vi "correction_data_starter.vi"() -> ()   [LabVIEW 2020]
uses:
  CasaoManagerGeneralSpecifications.ctl
  General dimensions definition.ctl
  Point2D.ctl
  Point2Df.ctl
  WavefrontCorrector.lvclass
  Camera.lvclass
  CorrectionDataManager.lvclass
  Image.lvclass
  InteractionMatrixAcquisitionParameters.ctl
  HasoSlopes.lvclass
  Data alignment enum.ctl
  InteractionMatrixToCommandMatrixParameters.ctl
panel:
  out "Camera Image (2N)":u32[][](graph)
  in  "Start Acq":bool
  out "Camera Image (2N+1)":u32[][](graph)
  in  "number of images to sum":u32=1
  in  "Exposure time (us)":i32=1000
  out "# of valid actuators":u32
  out "Singular values":dbl[](graph)
  in  "Correction data file name":string="Data\\data_correction_manager_example.aomi"
  in  "WavefrontCorrector Configuration file path":path
  out "error out":errorcluster
  out "Informations extracted \nfrom configuration files":T1 caption="Informations extracted from configuration files"
  in  "Haso configuration file path":path
  # "This example is Hardware-dependant, \nplease use your own Haso and corrector configuration file and acquisition system"
  # "Acquisition parameters"
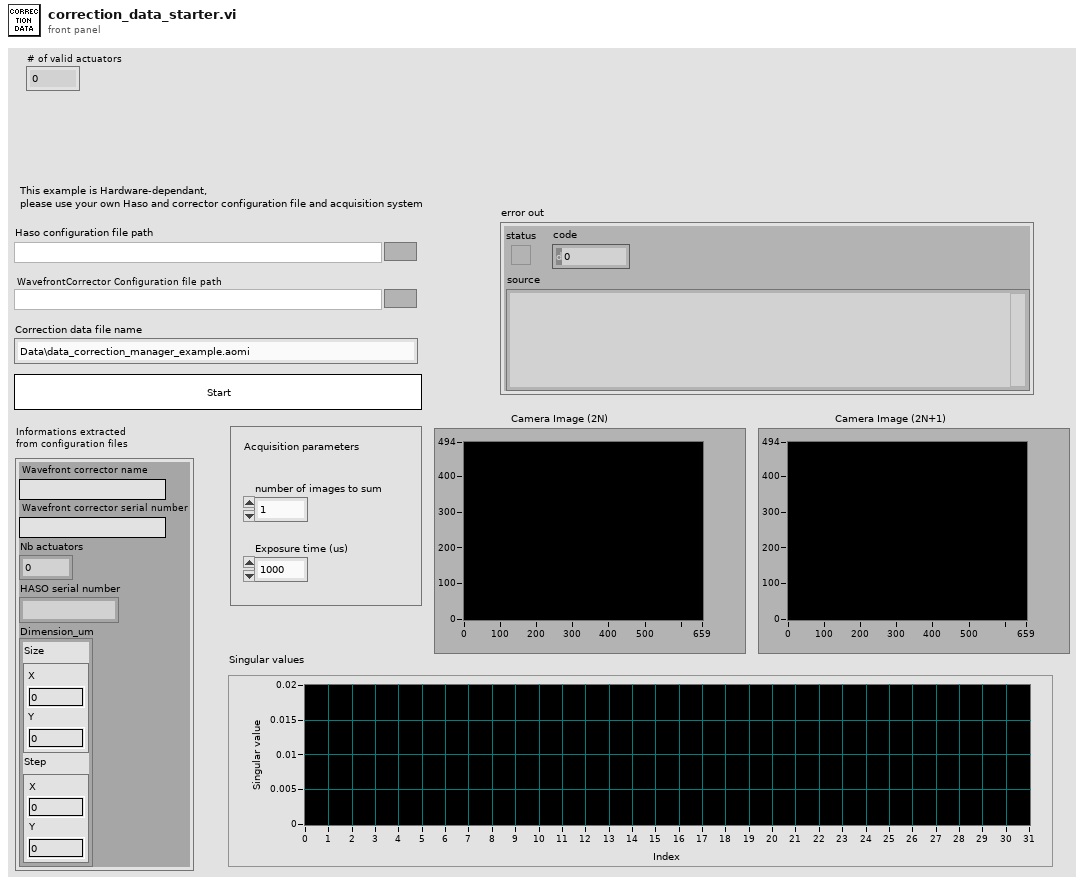
[diagram p1: front panel]
types:
  T1 = typedef "CasaoManagerGeneralSpecifications.ctl" = cluster{"Wavefront corrector name":string, "Wavefront corrector serial number":string, "Nb actuators":i32, "HASO serial number":string, "Dimension_um":T2}
  T2 = typedef "General dimensions definition.ctl" = cluster{"Size":T3, "Step":T4}
  T3 = typedef "Point2D.ctl" = cluster{"X":u32, "Y":u32}
  T4 = typedef "Point2Df.ctl" = cluster{"X":sgl, "Y":sgl}
  T5 = typedef "InteractionMatrixAcquisitionParameters.ctl" = cluster{"Push - Pull value":sgl}
  T6 = typedef "Data alignment enum.ctl" = enum16{"8", "16", "32"}
  T7 = typedef "InteractionMatrixToCommandMatrixParameters.ctl" = cluster{"Number of kept modes":i32, "Tilt filtering":bool}
  T8 = typedef "Wavefront Corrector states - ONE.ctl" = cluster{"Max":sgl, "Min":sgl, "Validity":enum16{"valid", "fixed", "invalid"}, "Fixed_Position":sgl}
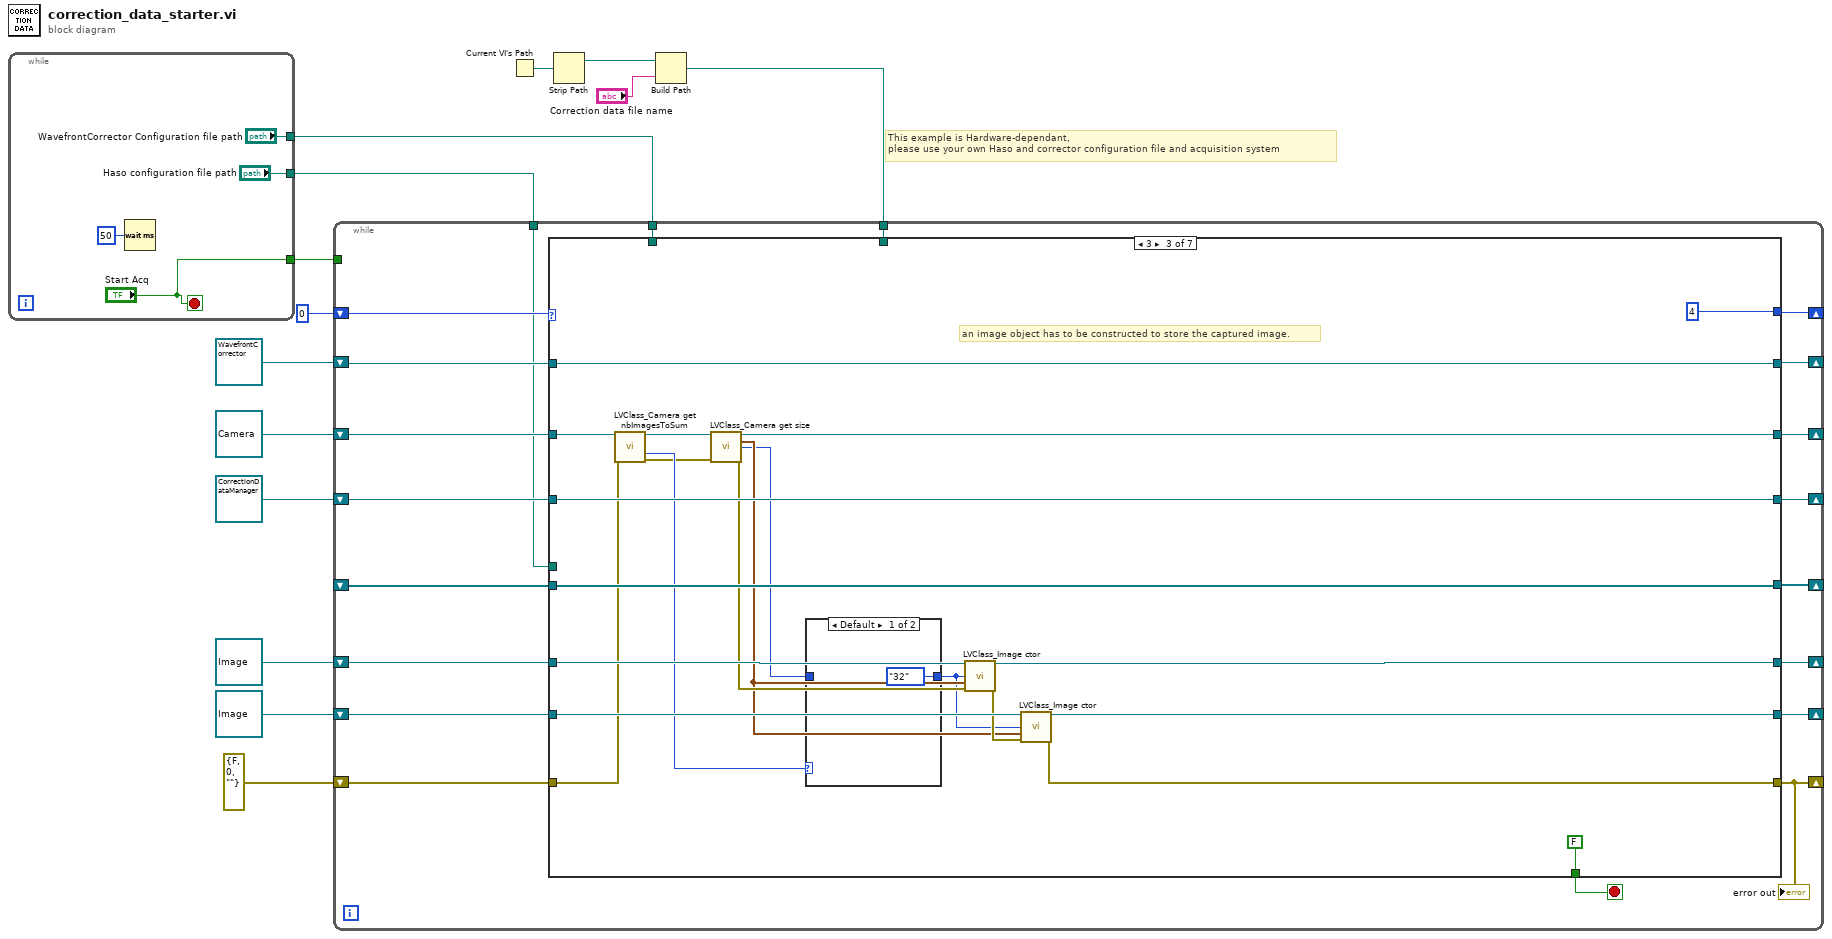
[diagram p0: block diagram]
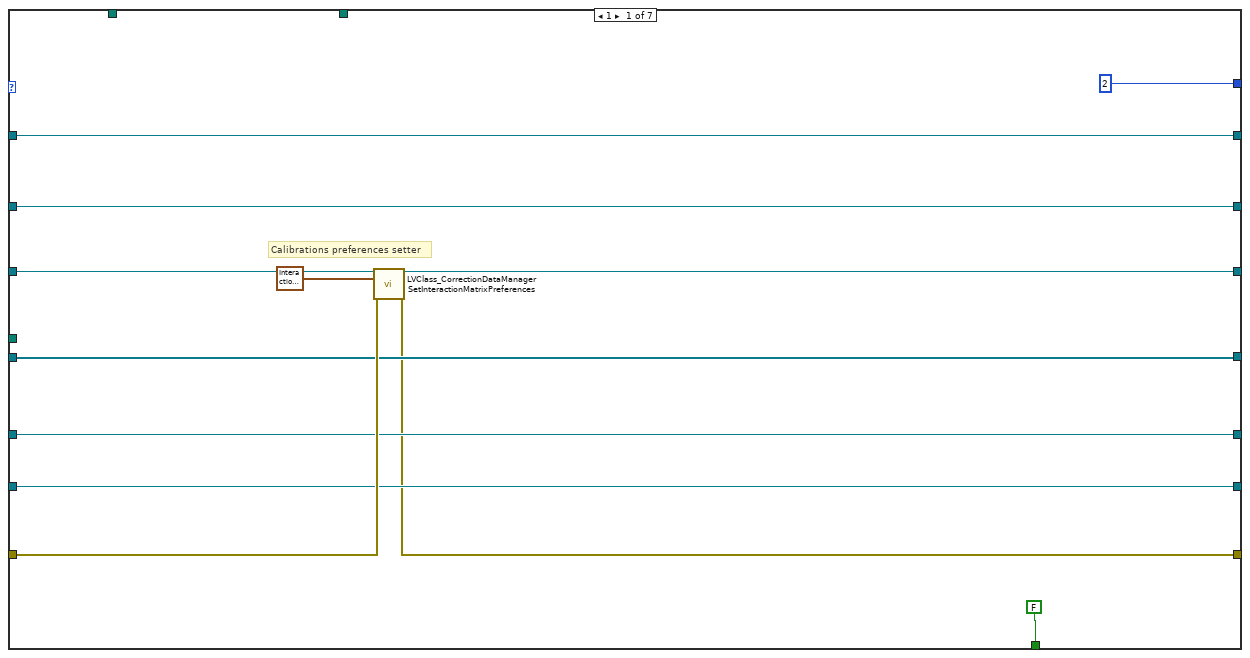
[diagram p2: hidden frame]
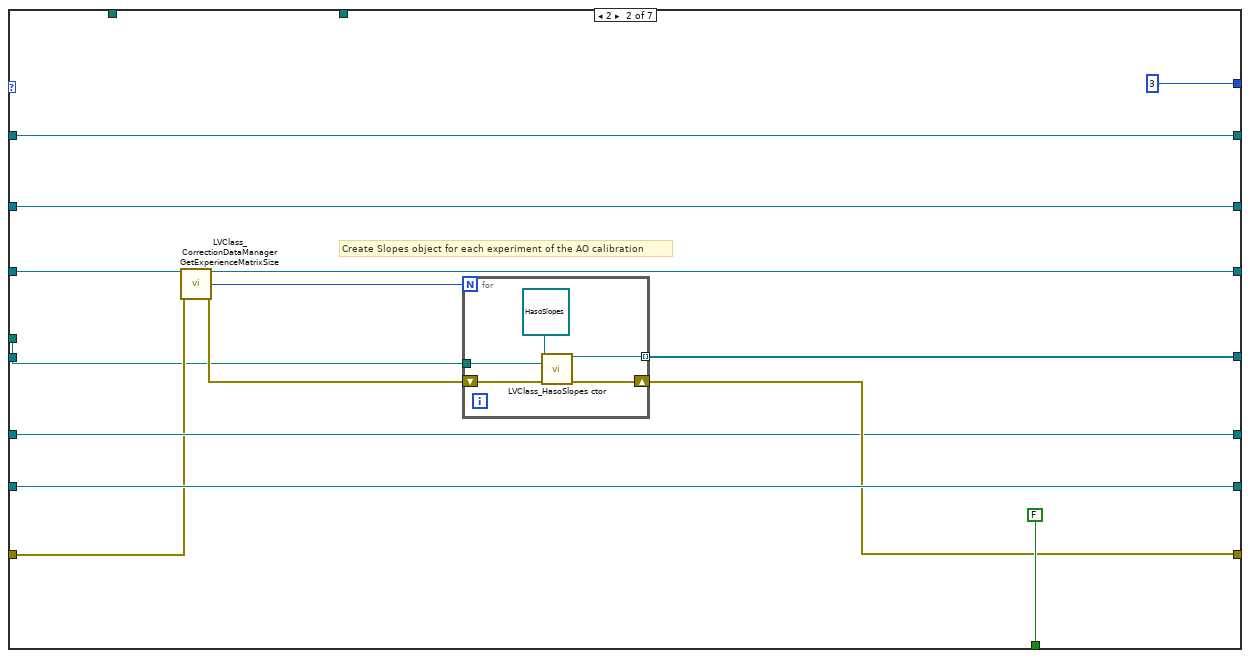
[diagram p3: hidden frame]
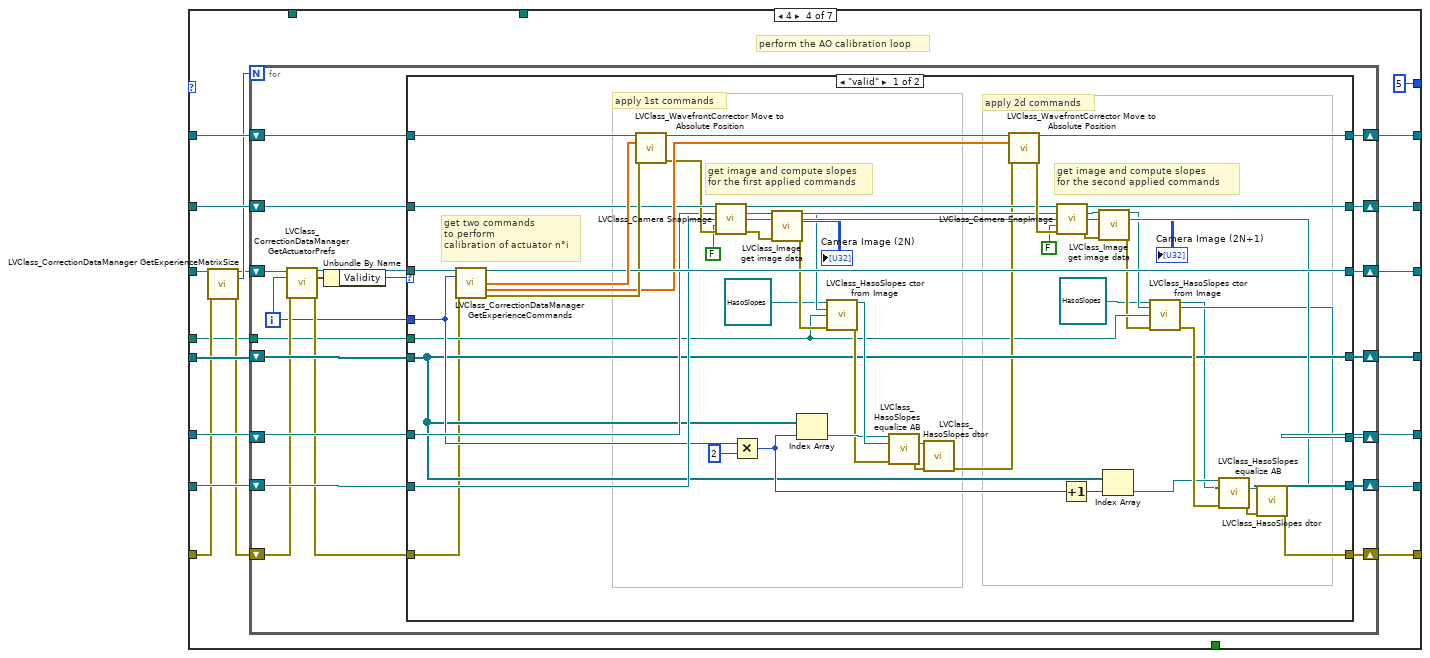
[diagram p5: hidden frame]
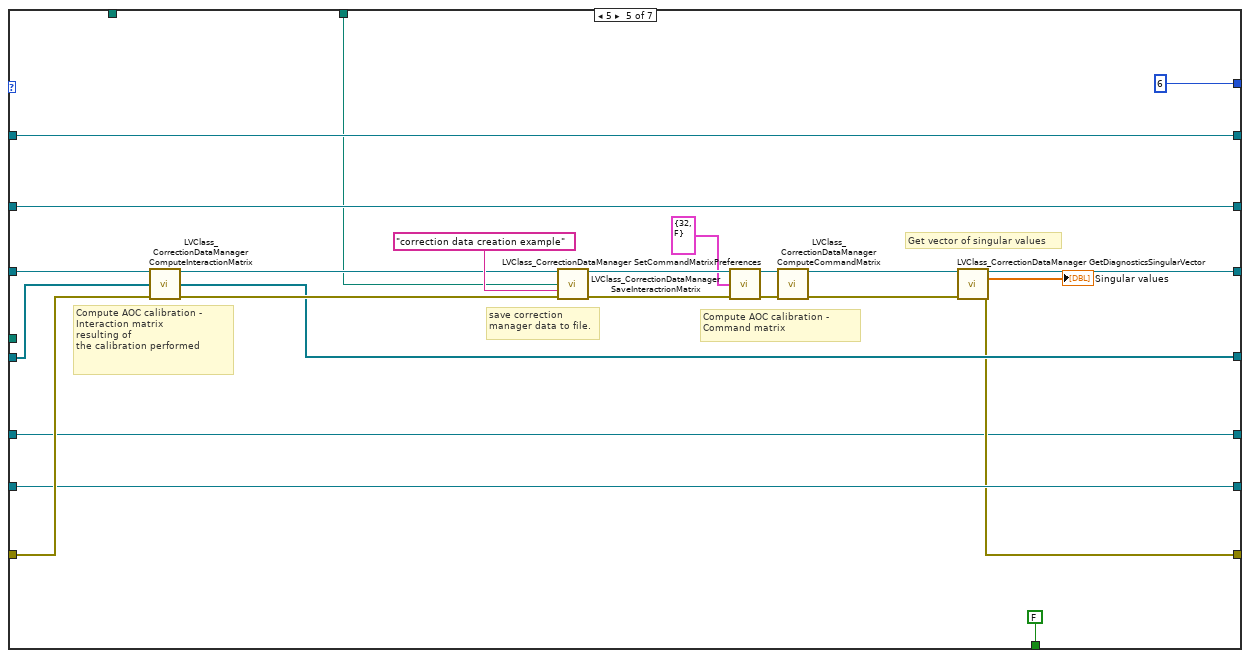
[diagram p7: hidden frame]
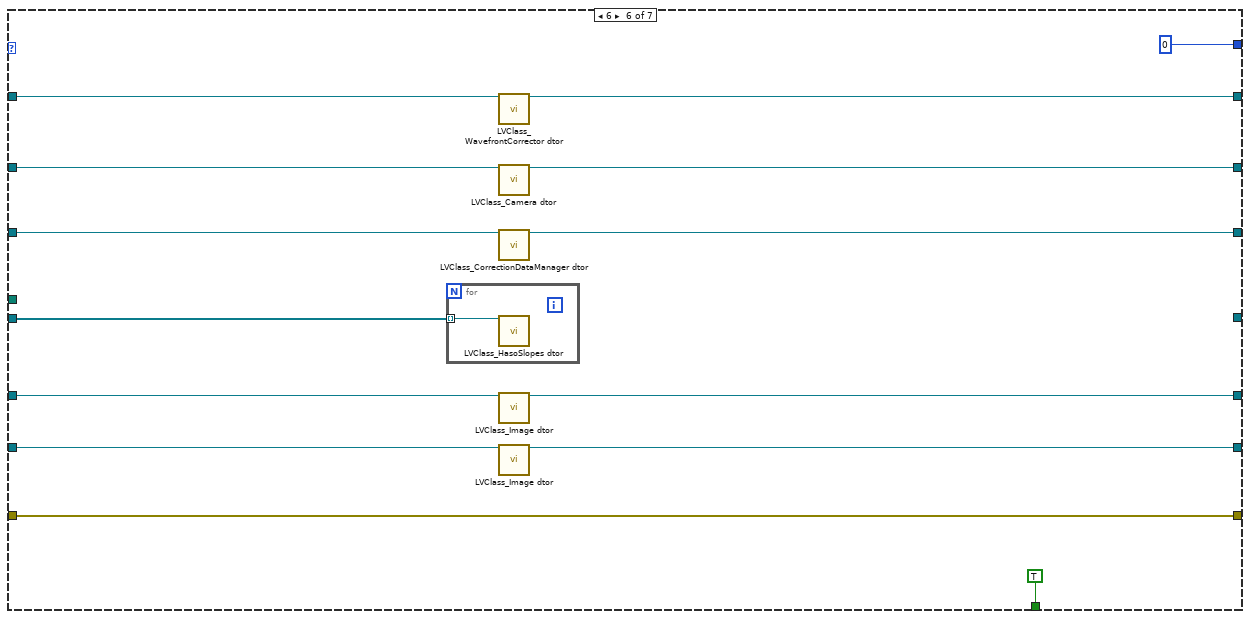
[diagram p8: hidden frame]
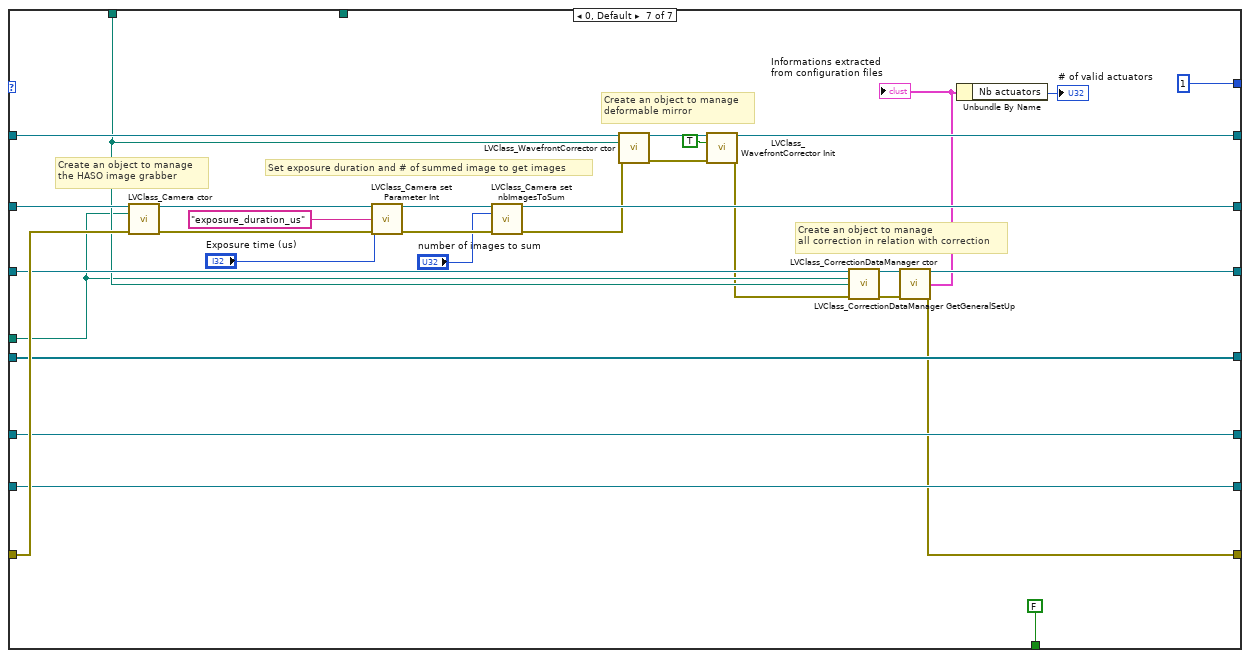
[diagram p9: hidden frame]
diagram:
  # "This example is Hardware-dependant, \nplease use your own Haso and corrector configuration file and acquisition system"
  n1 = while {
    tunnel: ["Start Acq"] -> w8
    tunnel: ["Haso configuration file path"] -> w2
    tunnel: ["WavefrontCorrector Configuration file path"] -> w1
    stop <- "Start Acq" stop-if-true
    n2 = Wait (ms)(milliseconds to wait=u32 50) -> ()  [unwired: 1 out]
  }
  n3 = Current VI's Path() -> (path=w5:path)
  n4 = Strip Path(path=w5) -> (stripped path=w7:path)  [unwired: 1 out]
  n5 = Build Path(base path=w7, name or relative path="Correction data file name") -> (appended path=w4:path)
  n6 = while {
    shift-right: [w30] -> _
    shift-left: refnum<class "WavefrontCorrector.lvclass"> refnum ("WavefrontCorrector in") -> [w32]
    shift-right: [w28] -> _
    shift-left: refnum<class "Camera.lvclass"> refnum ("Camera") -> [w35]
    shift-right: [w29] -> _
    shift-left: refnum<class "CorrectionDataManager.lvclass"> refnum ("CorrectionDataManager in") -> [w31]
    shift-right: [w25] -> _
    shift-left: refnum<class "Image.lvclass"> refnum ("Image in") -> [w27]
    shift-right: [w37] -> _
    shift-left: 0 -> [w38]
    shift-right: [w23] -> _
    shift-left: errorcluster {"status"=FALSE, "code"=0, "source"=""} ("error out") -> [w34]
    tunnel: w1 -> [w33]
    tunnel: w2 -> [w19]
    shift-right: [w26] -> _
    shift-left: _ -> [w24]
    shift-right: [w21] -> _
    shift-left: refnum<class "Image.lvclass"> refnum ("Image out") -> [w22]
    tunnel: w8 -> [_]
    tunnel: w4 -> [w20]
    stop <- w36 stop-if-true
    n7 = case shown="3" w38 {
      tunnel: [2 3 4 5 6 0 1] -> w37
      tunnel: [FALSE FALSE FALSE _ FALSE TRUE FALSE] -> w36
      tunnel: w35 -> [w43 w60 w76 w104 w193 w224 w256]
      tunnel: [w39 w58 w86 w105 w191 w214 w230] -> w23
      tunnel: w34 -> [w46 w55 w73 w95 w208 w214 w255]
      tunnel: w33 -> [_ _ _ _ _ _ w252]
      tunnel: w32 -> [w44 w61 w84 w110 w194 w223 w254]
      tunnel: w19 -> [_ w51 _ w93 _ _ w249]
      tunnel: w31 -> [w47 w53 w83 w98 w210 w220 w253]
      tunnel: [w44 w61 w84 w107 w194 w219 w245] -> w30
      tunnel: [w40 w52 w83 w106 w195 w213 w232] -> w29
      tunnel: [w43 w60 w85 w103 w193 w218 w242] -> w28
      tunnel: w27 -> [w42 w59 w88 w102 w192 w221 w250]
      tunnel: [w45 w62 w82 w108 w197 _ w251] -> w26
      tunnel: [w42 w59 w87 w99 w192 w217 w250] -> w25
      tunnel: w24 -> [w45 _ w82 w109 w209 w222 w251]
      tunnel: w22 -> [w41 w57 w81 w101 w190 w216 w248]
      tunnel: [w41 w57 w80 w100 w190 w215 w248] -> w21
      tunnel: w20 -> [_ _ _ _ w189 _ _]
      frame 1 {
        # "Calibrations preferences setter"
        n8 = call "LVClass_CorrectionDataManager SetInteractionMatrixPreferences.vi"("CorrectionDataManager in"=w47, "push_pull_value"=T5 {"Push - Pull value"=0.2} ("Interaction Matrix Parameters 2"), "error in (no error)"=w46) -> ("CorrectionDataManager out"=w40:refnum<class "CorrectionDataManager.lvclass">, "error out"=w39:errorcluster)  [unwired: 11 in]
      }
      frame 2 {
        # "Create Slopes object for each experiment of the AO calibration"
        n9 = call "LVClass_CorrectionDataManager GetExperienceMatrixSize.vi"("CorrectionDataManager in"=w53, "error in (no error)"=w55) -> ("CorrectionDataManager out"=w52:refnum<class "CorrectionDataManager.lvclass">, "# of experiments"=w56:u32, "error out"=w54:errorcluster)  [unwired: 10 in, 1 out]
        n10 = for {
          N: w56 -> [_]
          tunnel: w51 -> [w69]
          tunnel: [w67] -> w62 mode=indexing
          shift-right: [w66] -> w58
          shift-left: w54 -> [w65]
          n11 = call "LVClass_HasoSlopes ctor.vi"("HasoSlopes in"=refnum<class "HasoSlopes.lvclass"> refnum, "Configuration file path"=w69, "error in (no error)"=w65) -> ("HasoSlopes out"=w67:refnum<class "HasoSlopes.lvclass">, "error out"=w66:errorcluster)  [unwired: 11 in]
        }
      }
      frame 3 {
        # "an image object has to be constructed to store the captured image."
        n12 = call "LVClass_Camera get nbImagesToSum.vi"("Camera in"=w76, "error in (no error)"=w73) -> ("Camera out"=w75:refnum<class "Camera.lvclass">, "nb_image"=w74:u32, "error out"=w72:errorcluster)  [unwired: 11 in]
        n13 = call "LVClass_Camera get size.vi"("Camera in"=w75, "error in (no error)"=w72) -> ("Camera out"=w85:refnum<class "Camera.lvclass">, "size"=w77:T3, "Number of bits"=w71:T6, "error out"=w79:errorcluster)  [unwired: 10 in]
        n14 = case shown="Default" w74 {
          tunnel: [Data_alignment_enum."32" ("Number of bits") w92] -> w70
          tunnel: w71 -> [_ w92]
          frame Default {
          }
          frame 1 {
          }
        }
        n15 = call "LVClass_Image ctor.vi"("Image in"=w81, "Data alignment"=w70, "Size"=w77, "error in (no error)"=w79) -> ("Image out"=w80:refnum<class "Image.lvclass">, "error out"=w78:errorcluster)  [unwired: 10 in]
        n16 = call "LVClass_Image ctor.vi"("Image in"=w88, "Data alignment"=w70, "Size"=w77, "error in (no error)"=w78) -> ("Image out"=w87:refnum<class "Image.lvclass">, "error out"=w86:errorcluster)  [unwired: 10 in]
      }
      frame 4 {
        # "perform the AO calibration loop"
        n17 = call "LVClass_CorrectionDataManager GetExperienceMatrixSize.vi"("CorrectionDataManager in"=w98, "error in (no error)"=w95) -> ("CorrectionDataManager out"=w96:refnum<class "CorrectionDataManager.lvclass">, "# of valid actuators"=w97:u32, "error out"=w94:errorcluster)  [unwired: 10 in, 1 out]
        n18 = for {
          N: w97 -> [_]
          shift-right: [w130] -> w106
          shift-left: w96 -> [w129]
          shift-right: [w125] -> w107
          shift-left: w110 -> [w131]
          shift-right: [w124] -> w105
          shift-left: w94 -> [w117]
          shift-right: [w122] -> w103
          shift-left: w104 -> [w123]
          shift-right: [w119] -> w100
          shift-left: w101 -> [w120]
          shift-right: [w118] -> w99
          shift-left: w102 -> [w121]
          shift-right: [w126] -> w108
          shift-left: w109 -> [w127]
          tunnel: w93 -> [w112]
          i -> [w113]
          n19 = call "LVClass_CorrectionDataManager GetActuatorPrefs.vi"("CorrectionDataManager in"=w129, "N° actuator"=w113, "error in (no error)"=w117) -> ("CorrectionDataManager out"=w128:refnum<class "CorrectionDataManager.lvclass">, "Actuator state"=w116:T8, "error out"=w115:errorcluster)  [unwired: 10 in]
          n20 = Unbundle By Name(w116) -> ("Validity"=w114:enum16{"valid", "fixed", "invalid"})
          n21 = case shown="\"valid\"" w114 {
            tunnel: w131 -> [w181 w188]
            tunnel: [w179 w183] -> w130
            tunnel: w128 -> [w178 w183]
            tunnel: w127 -> [w146 w184]
            tunnel: [w146 w184] -> w126
            tunnel: [w173 w188] -> w125
            tunnel: [w135 w182] -> w124
            tunnel: w123 -> [w172 w187]
            tunnel: [w168 w187] -> w122
            tunnel: w121 -> [w166 w185]
            tunnel: w120 -> [w167 w186]
            tunnel: [w140 w186] -> w119
            tunnel: [w162 w185] -> w118
            tunnel: w115 -> [w132 w182]
            tunnel: w112 -> [w139 _]
            tunnel: w113 -> [w147 _]
            frame "valid" {
              # "apply 2d commands"
              # "apply 1st commands"
              # "get image and compute slopes\nfor the second applied commands"
              # "get image and compute slopes\nfor the first applied commands"
              # "get two commands\nto perform \ncalibration of actuator n°i"
              n22 = call "LVClass_CorrectionDataManager GetExperienceCommands.vi"("CorrectionDataManager in"=w178, "N° actuator"=w147, "error in (no error)"=w132) -> ("CorrectionDataManager out"=w179:refnum<class "CorrectionDataManager.lvclass">, "First DeltaCommand"=w180:sgl[], "Second DeltaCommand"=w175:sgl[], "error out"=w177:errorcluster)  [unwired: 9 in]
              n23 = call "LVClass_WavefrontCorrector Move to Absolute Position.vi"("WavefrontCorrector in"=w181, "Absolute Positions"=w180, "error in (no error)"=w177) -> ("WavefrontCorrector out"=w176:refnum<class "WavefrontCorrector.lvclass">, "error out"=w171:errorcluster)  [unwired: 11 in]
              n24 = call "LVClass_Camera SnapImage.vi"("Camera in"=w172, "Image"=w167, "Image RAW"=w166, "remove_background"=FALSE, "error in (no error)"=w171) -> ("Camera out"=w169:refnum<class "Camera.lvclass">, "Image (dup)"=w151:refnum<class "Image.lvclass">, "Image (dup) RAW"=w164:refnum<class "Image.lvclass">, "error out"=w149:errorcluster)  [unwired: 7 in]
              n25 = Multiply(x=w147, y=2) -> (x*y=w156:i32)
              n26 = call "LVClass_Image get image data.vi"("Image in"=w151, "error in (no error)"=w149) -> ("Image out"=w142:refnum<class "Image.lvclass">, "Image data out"=→"Camera Image (2N)":u32[][], "error out"=w150:errorcluster)  [unwired: 11 in]
              n27 = Index Array(array=w146, index=w156) -> (element=w155:refnum<class "HasoSlopes.lvclass">)
              n28 = call "LVClass_HasoSlopes ctor from Image.vi"("HasoSlopes in"=refnum<class "HasoSlopes.lvclass"> refnum, "Image.lvclass"=w142, "Haso configuration file"=w139, "error in (no error)"=w150) -> ("HasoSlopes out"=w159:refnum<class "HasoSlopes.lvclass">, "error out"=w148:errorcluster)  [unwired: 10 in]
              n29 = call "LVClass_HasoSlopes equalize AB.vi"("HasoSlopes dest in"=w155, "HasoSlopes source in"=w159, "error in (no error)"=w148) -> ("HasoSlopes source out"=w158:refnum<class "HasoSlopes.lvclass">, "error out"=w145:errorcluster)  [unwired: 10 in, 1 out]
              n30 = call "LVClass_HasoSlopes dtor.vi"("HasoSlopes in"=w158, "error in (no error)"=w145) -> ("error out"=w144:errorcluster)  [unwired: 12 in, 1 out]
              n31 = call "LVClass_WavefrontCorrector Move to Absolute Position.vi"("WavefrontCorrector in"=w176, "Absolute Positions"=w175, "error in (no error)"=w144) -> ("WavefrontCorrector out"=w173:refnum<class "WavefrontCorrector.lvclass">, "error out"=w170:errorcluster)  [unwired: 11 in]
              n32 = call "LVClass_Camera SnapImage.vi"("Camera in"=w169, "Image"=w151, "Image RAW"=w164, "remove_background"=FALSE, "error in (no error)"=w170) -> ("Camera out"=w168:refnum<class "Camera.lvclass">, "Image (dup)"=w141:refnum<class "Image.lvclass">, "Image (dup) RAW"=w162:refnum<class "Image.lvclass">, "error out"=w137:errorcluster)  [unwired: 7 in]
              n33 = Increment(x=w156) -> (x+1=w154:i32)
              n34 = call "LVClass_Image get image data.vi"("Image in"=w141, "error in (no error)"=w137) -> ("Image out"=w140:refnum<class "Image.lvclass">, "Image data out"=→"Camera Image (2N+1)":u32[][], "error out"=w136:errorcluster)  [unwired: 11 in]
              n35 = Index Array(array=w146, index=w154) -> (element=w153:refnum<class "HasoSlopes.lvclass">)
              n36 = call "LVClass_HasoSlopes ctor from Image.vi"("HasoSlopes in"=refnum<class "HasoSlopes.lvclass"> refnum, "Image.lvclass"=w140, "Haso configuration file"=w139, "error in (no error)"=w136) -> ("HasoSlopes out"=w138:refnum<class "HasoSlopes.lvclass">, "error out"=w174:errorcluster)  [unwired: 10 in]
              n37 = call "LVClass_HasoSlopes equalize AB.vi"("HasoSlopes dest in"=w153, "HasoSlopes source in"=w138, "error in (no error)"=w174) -> ("HasoSlopes source out"=w157:refnum<class "HasoSlopes.lvclass">, "error out"=w143:errorcluster)  [unwired: 10 in, 1 out]
              n38 = call "LVClass_HasoSlopes dtor.vi"("HasoSlopes in"=w157, "error in (no error)"=w143) -> ("error out"=w135:errorcluster)  [unwired: 12 in, 1 out]
            }
            frame "fixed", Default {
            }
          }
        }
      }
      frame 5 {
        # "Compute AOC calibration - Interaction matrix\nresulting of\nthe calibration performed"
        # "Compute AOC calibration - Command matrix"
        # "Get vector of singular values"
        # "save correction\nmanager data to file."
        n39 = call "LVClass_CorrectionDataManager ComputeInteractionMatrix.vi"("CorrectionDataManager in"=w210, "HasoSlopes array"=w209, "error in (no error)"=w208) -> ("CorrectionDataManager out"=w199:refnum<class "CorrectionDataManager.lvclass">, "HasoSlopes array 2"=w197:refnum<class "HasoSlopes.lvclass">[], "error out"=w198:errorcluster)  [unwired: 10 in]
        n40 = call "LVClass_CorrectionDataManager SaveInteractrionMatrix.vi"("CorrectionDataManager in"=w199, "Interaction Matrix file path"=w189, "comment"="correction data creation example", "error in (no error)"=w198) -> ("CorrectionDataManager out"=w203:refnum<class "CorrectionDataManager.lvclass">, "error out"=w200:errorcluster)  [unwired: 10 in]
        n41 = call "LVClass_CorrectionDataManager SetCommandMatrixPreferences.vi"("CorrectionDataManager in"=w203, "Prefs"=T7 {"Number of kept modes"=32, "Tilt filtering"=FALSE}, "error in (no error)"=w200) -> ("CorrectionDataManager out"=w204:refnum<class "CorrectionDataManager.lvclass">, "error out"=w207:errorcluster)  [unwired: 11 in]
        n42 = call "LVClass_CorrectionDataManager ComputeCommandMatrix.vi"("CorrectionDataManager in"=w204, "error in (no error)"=w207) -> ("CorrectionDataManager out"=w205:refnum<class "CorrectionDataManager.lvclass">, "error out"=w206:errorcluster)  [unwired: 12 in]
        n43 = call "LVClass_CorrectionDataManager GetDiagnosticsSingularVector.vi"("CorrectionDataManager in"=w205, "error in (no error)"=w206) -> ("CorrectionDataManager out"=w195:refnum<class "CorrectionDataManager.lvclass">, "ArrayOfSingularValues"=→"Singular values":dbl[], "error out"=w191:errorcluster)  [unwired: 11 in]
      }
      frame 6 {
        n44 = for {
          tunnel: w222 -> [w227] mode=indexing
          n45 = call "LVClass_HasoSlopes dtor.vi"("HasoSlopes in"=w227) -> ()  [unwired: 13 in, 2 out]
        }
        n46 = call "LVClass_WavefrontCorrector dtor.vi"("WavefrontCorrector in"=w223) -> ("WavefrontCorrector out"=w219:refnum<class "WavefrontCorrector.lvclass">)  [unwired: 13 in, 1 out]
        n47 = call "LVClass_Camera dtor.vi"("Camera in"=w224) -> ("Camera out"=w218:refnum<class "Camera.lvclass">)  [unwired: 13 in, 1 out]
        n48 = call "LVClass_CorrectionDataManager dtor.vi"("CorrectionDataManager in"=w220) -> ("CorrectionDataManager out"=w213:refnum<class "CorrectionDataManager.lvclass">)  [unwired: 13 in, 1 out]
        n49 = call "LVClass_Image dtor.vi"("Image in"=w216) -> ("Image out"=w215:refnum<class "Image.lvclass">)  [unwired: 13 in, 1 out]
        n50 = call "LVClass_Image dtor.vi"("Image in"=w221) -> ("Image out"=w217:refnum<class "Image.lvclass">)  [unwired: 13 in, 1 out]
      }
      frame 0, Default {
        # "Create an object to manage \nall correction in relation with correction"
        # "Set exposure duration and # of summed image to get images"
        # "Create an object to manage \ndeformable mirror"
        # "Create an object to manage \nthe HASO image grabber"
        n51 = call "LVClass_Camera ctor.vi"("Camera"=w256, "Configuration file path"=w249, "error in (no error)"=w255) -> ("Camera (new)"=w237:refnum<class "Camera.lvclass">, "error out"=w236:errorcluster)  [unwired: 11 in]
        n52 = call "LVClass_Camera set Parameter Int.vi"("Camera in"=w237, "parameter_name"="exposure_duration_us", "value"="Exposure time (us)", "error in (no error)"=w236) -> ("Camera out"=w243:refnum<class "Camera.lvclass">, "error out"=w241:errorcluster)  [unwired: 10 in]
        n53 = call "LVClass_Camera set nbImagesToSum.vi"("Camera in"=w243, "nb_image"="number of images to sum", "error in (no error)"=w241) -> ("Camera out"=w242:refnum<class "Camera.lvclass">, "error out"=w235:errorcluster)  [unwired: 11 in]
        n54 = call "LVClass_WavefrontCorrector ctor.vi"("WavefrontCorrector in"=w254, "PathToWavefrontCorrectorSetupFile"=w252, "error in (no error)"=w235) -> ("WavefrontCorrector out"=w246:refnum<class "WavefrontCorrector.lvclass">, "error out"=w244:errorcluster)  [unwired: 11 in]
        n55 = call "LVClass_WavefrontCorrector Init.vi"("WavefrontCorrector in"=w246, "set_init_state_from_config_file"=TRUE, "error in (no error)"=w244) -> ("WavefrontCorrector out"=w245:refnum<class "WavefrontCorrector.lvclass">, "error out"=w234:errorcluster)  [unwired: 11 in]
        n56 = call "LVClass_CorrectionDataManager ctor.vi"("CorrectionDataManager in"=w253, "PathTohaso_config_file_path"=w249, "PathTowfc_config_file_path"=w252, "error in (no error)"=w234) -> ("CorrectionDataManager out"=w233:refnum<class "CorrectionDataManager.lvclass">, "error out"=w231:errorcluster)  [unwired: 10 in]
        n57 = call "LVClass_CorrectionDataManager GetGeneralSetUp.vi"("CorrectionDataManager in"=w233, "error in (no error)"=w231) -> ("CorrectionDataManager out"=w232:refnum<class "CorrectionDataManager.lvclass">, "general"=w228:T1, "error out"=w230:errorcluster)  [unwired: 11 in]
        "Informations extracted \nfrom configuration files" <- w228
        n58 = Unbundle By Name(w228) -> ("Nb actuators"=→"# of valid actuators":i32)
      }
    }
    "error out" <- w23
  }
